vi "Create.vi"(8 "error in (no error)":errorcluster) -> (0 "error out":errorcluster, 3 "CT-De-energize-Cmd.lvclass":refnum<class "CT-De-energize-Cmd.lvclass">)   [LabVIEW 2013, in "CT-De-energize-Cmd.lvclass"]
uses:
  CT-De-energize-Cmd.lvclass
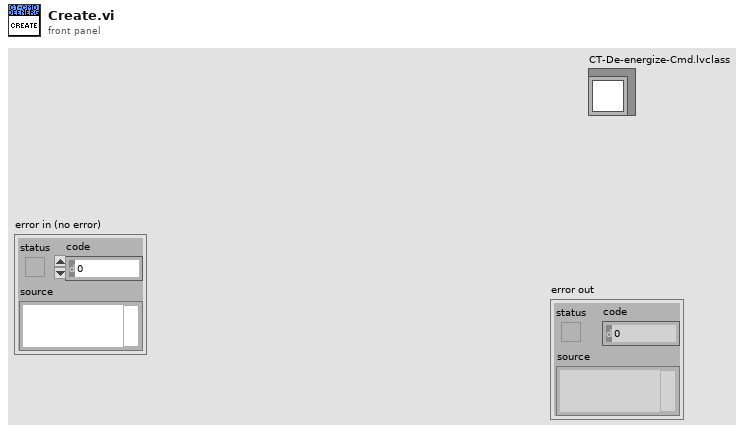
[diagram p1: front panel]
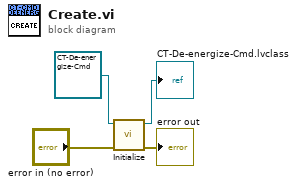
[diagram p0: block diagram]
diagram:
  n1 = call-dynamic "Initialize.vi"("error in (no error)"="error in (no error)", "CT-De-energize-Cmd in"=refnum<class "CT-De-energize-Cmd.lvclass"> refnum ("CT-De-energize-Cmd.lvclass")) -> ("error out"=→"error out":errorcluster, "CT-De-energize-Cmd out"=→"CT-De-energize-Cmd.lvclass":refnum<class "CT-De-energize-Cmd.lvclass">)  [unwired: 8 in]
